vi "Create.vi"(8 "error in (no error)":errorcluster, 10 "Starting Values (Empty)":map{string[], T1}(c390)) -> (0 "error out":errorcluster, 3 "Tree Map out":refnum<class "Tree Map.lvclass">)   [LabVIEW 2020, in "VI Properties Editor.lvlib" / "VI Properties Tree Map.lvlib" / "Tree Map.lvclass"]
uses:
  Tree Map.lvclass
  Tree Map.lvclass/Tree Map.ctl
  Tree Entry.ctl
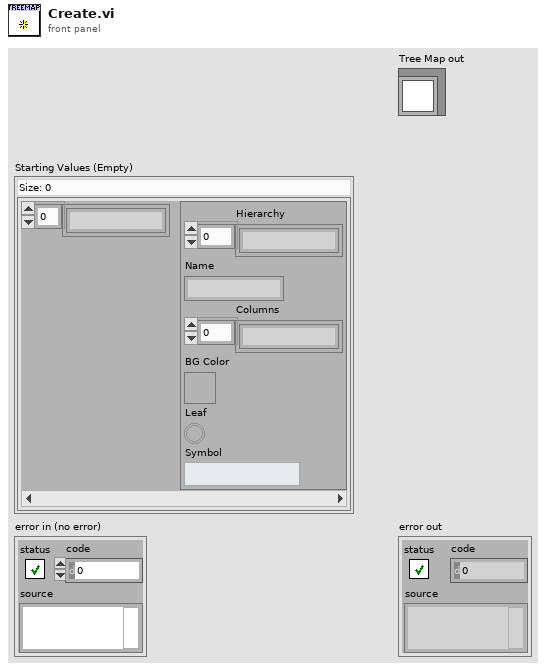
[diagram p1: front panel]
types:
  T1 = typedef "VI Properties Editor.lvlib/VI Properties Tree Map.lvlib/Tree Map.lvclass/Tree Entry.ctl" = cluster{"Hierarchy":string[], "Name":string, "Columns":string[], "BG Color":u32, "Leaf":bool, "Symbol":string}
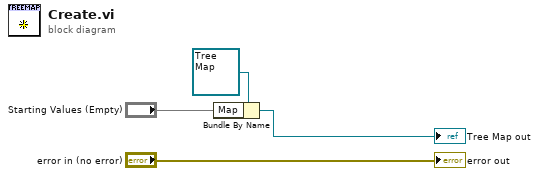
[diagram p0: block diagram]
diagram:
  n1 = Bundle By Name(cluster=refnum<class "Tree Map.lvclass"> refnum ("Tree Map in"), "Map"="Starting Values (Empty)") -> (→"Tree Map out":refnum<class "Tree Map.lvclass">)
  "error out" <- "error in (no error)"
